vi "HFRR ADV v04.vi"() -> ()   [LabVIEW 2025] (continued)
                n419 = Array To Spreadsheet String(delimiter (Tab)=";", array=w743, 3:"" ("format string")) -> (spreadsheet string=w745:string)
                "String 9" <- w745
                n420 = Concatenate Strings("FF ( V ); DP( mincron ) " ("character string"), "\r") -> (w758:string)
                n421 = local read "file count"() -> (w741:i32)
                n422 = local read "FILE 2"() -> (w746:string)
                n423 = local write "save dpt"(FALSE ("Hold 3")) -> ()
                n424 = Number To Decimal String(number=w741) -> (decimal integer string=w747:string)  [unwired: 1 in]
                n425 = Concatenate Strings(w746, w747) -> (w739:string)
                n426 = Concatenate Strings("C:\\LAB-IQ-NXT\\data" ("Substring"), w739) -> (w754:string)
                n427 = Concatenate Strings(w754, ".dpf" ("Substring")) -> (w752:string)
                n428 = Add(x=1, y=w741) -> (x+y=w742:i32)
                n429 = local write "file count"(w742) -> ()
                n430 = String To Path(string=w752) -> (path=w750:path)
                n431 = call <vilib>:"Write Characters To File.vi"("append to file? (new file:F)"=FALSE, "character string"=w758, "file path (dialog if empty)"=w750) -> ("new file path (Not A Path if cancelled)"=w755:path)  [unwired: 2 in]
                n432 = call <vilib>:"Write Characters To File.vi"("append to file? (new file:F)"=TRUE, "character string"=w745, "file path (dialog if empty)"=w755) -> ()  [unwired: 2 in, 1 out]
              }
            }
          }
          frame #5 {
            n433 = case shown="True" "Hold 4" {
              frame False {
              }
              frame True {
                n434 = File Dialog(6:"*.dpf" ("pattern"), 11:path "C:/LAB-IQ-NXT" ("start path")) -> (0:w765:errorcluster, 3:w780:path)  [unwired: 5 in, 2 out]
                n435 = Unbundle(w765) -> ()  [unwired: 3 out]
                n436 = call <vilib>:"Read Characters From File.vi"("file path (dialog if empty)"=w780) -> ("character string"=w770:string)  [unwired: 5 in, 3 out]
                n437 = Spreadsheet String To Array(delimiter (Tab)=";", format string="%S", spreadsheet string=w770, array type (2D Dbl)=string[][] []) -> (array=w774:string[][])
                n438 = for {
                  tunnel: w774 -> [w784] mode=indexing
                  tunnel: [w783] -> w775 mode=indexing
                  n439 = for {
                    tunnel: w784 -> [w786] mode=indexing
                    tunnel: [w785] -> w783 mode=indexing
                    n440 = call <vilib>:"Trim Whitespace.vi"("string"=w786) -> ("trimmed string"=w785:string)  [unwired: 1 in]
                  }
                }
                n441 = Fract/Exp String To Number(string=w775) -> (number=w777:dbl[][])  [unwired: 3 in, 1 out]
                n442 = Array Subset(array=w777, index (row)=1 ("index (col)")) -> (w779:dbl[][])  [unwired: 3 in]
                n443 = Index Array(array=w779, index (col) #1=0 ("disabled index (col)"), index (col) #2=1 ("disabled index (col)")) -> (element #1=w768:dbl[], element #2=w767:dbl[])  [unwired: 2 in]
                n444 = Build Array(w768, w767) -> (→"Waveform Graph":dbl[][])
              }
            }
          }
        }
      }
      frame Error {
        w802 = u16 0 items=["None", "XON/XOFF", "RTS/CTS", "XON/XOFF & RTS/CTS", "DTR/DSR", "XON/XOFF & DTR/DSR"] ("flow control (0:none)  2")
        w800 = u16 10 items=["1.0"=10, "1.5"=15, "2.0"=20] ("stop bits 2")
        w798 = u16 0 items=["None", "Odd", "Even", "Mark", "Space"] ("parity 2")
        w799 = u32 10000  # timeout (10sec)
        n445 = VISA Close(VISA resource name=w794, error in (no error)=w791) -> (error out=w795:errorcluster)
        n446 = local read "Com Port 1"() -> (w787:refnum<visa-resource-name>)
        n447 = call <vilib>:"Clear Errors.vi"("error in (no error)"=w795) -> ("error out"=w792:errorcluster)  [unwired: 5 in, 1 out]
        n448 = local write "Sps 3"(0.0 ("Sps 4")) -> ()
        n449 = call-poly "VISA Configure Serial Port"("VISA resource name"=w787, "timeout (10sec)"=w799, "baud rate (9600)"=u32 250000 ("baud rate  2"), "data bits (8)"=u16 8 ("data bits  2"), "parity (0:none)"=w798, "error in (no error)"=w792, "stop bits (10: 1 bit)"=w800, "flow control (0:none)"=w802) -> ("VISA resource name out"=w803:refnum<visa-resource-name>, "error out"=w804:errorcluster)  [unwired: 6 in]
        n450 = flat-sequence {
          tunnel: w803 -> [w806]
          tunnel: w804 -> [w805]
          tunnel: [w806] -> w796
          tunnel: [w805] -> w788
          frame #0 {
            n451 = Wait (ms)(milliseconds to wait=u32 50) -> ()  [unwired: 1 out]
          }
        }
        "Residual Uno" <- ""
        "Port 1 Error" <- w788
      }
    }
    n452 = local read "Port 1a"() -> (w449:bool)
    n453 = local read "Port 3"() -> (w450:bool)
    n454 = Or(x=w450, y=w449) -> (x .or. y?=w452:bool)
    n455 = case shown="False" w452 {
      frame False {
        w463 = FALSE ("Visible")
        n456 = property on="Port 1a" class="Bool (strict)"("Visible"=w463) -> ()  [unwired: 2 in, 2 out]
        n457 = property on="Port 3" class="Bool (strict)"("Visible"=w463) -> ()  [unwired: 2 in, 2 out]
      }
      frame True {
        w464 = TRUE ("Visible")
        n458 = property on="Port 1a" class="Bool (strict)"("Visible"=w464) -> ()  [unwired: 2 in, 2 out]
        n459 = property on="Port 3" class="Bool (strict)"("Visible"=w464) -> ()  [unwired: 2 in, 2 out]
      }
    }
    n460 = local read "EXIT"() -> (w454:bool)
    "Error Uno" <- w448
  }
  n461 = while {
    tunnel: w43 -> [_]
    tunnel: [w829] -> _
    tunnel: w15 -> [_]
    tunnel: ["EXIT"] -> w40
    i -> [w829]
    stop <- "EXIT" stop-if-true
    # "C:\\LAB-IQ-NXT\\Scar View.exe"
    n462 = local read "RUN"() -> (w827:bool)
    n463 = local read "EDIT 2"() -> (w814:bool)
    n464 = case shown="False" w827 {
      frame False {
        n465 = local read "stopT"() -> (w1697:bool)
        n466 = case shown="True" w1697 {
          frame False {
          }
          frame True {
            w1698 = FALSE
            n467 = local write "st enable"(w1698) -> ()
            n468 = local write "stopT"(w1698) -> ()
          }
        }
      }
      frame True {
        "stopT" <- TRUE
      }
    }
    n469 = case shown="True" w814 {
      frame False {
        n470 = local write "Password 2"("" ("Password")) -> ()
        n471 = property on="Password 2" class="Str"("Visible"=FALSE) -> ()  [unwired: 2 in, 2 out]
      }
      frame True {
        n472 = property on="Password 2" class="Str"("Visible"=TRUE) -> ()  [unwired: 2 in, 2 out]
        n473 = Equal?(x="Password 2", y="HFRR1234") -> (x = y?=w842:bool)
        n474 = case shown="True" w842 {
          tunnel: "Password 2" -> [w845 _]
          frame False {
            n475 = String Length(string=w845) -> (length=w846:i32)
            n476 = Greater Than 0?(x=w846) -> (x > 0?=w844:bool)
            n477 = case shown="False" w844 {
              frame False {
                n478 = property on="Password 2" class="Str"("Caption.Text"="Password (Advance Setting)") -> ()  [unwired: 2 in, 2 out]
              }
              frame True {
                n479 = property on="Password 2" class="Str"("Caption.Text"="Incorrect Password!") -> ()  [unwired: 2 in, 2 out]
              }
            }
          }
          frame True {
            n480 = local write "Password 2"("" ("Password")) -> ()
            n481 = local write "Main Tab"(T2."Advance" ("Main Tab")) -> ()
            n482 = local write "EDIT 2"(FALSE ("EDIT 2")) -> ()
          }
        }
      }
    }
    n483 = Wait (ms)(milliseconds to wait=u32 50) -> ()  [unwired: 1 out]
    n484 = case shown="True" "EDIT 3" {
      frame False {
      }
      frame True {
        n485 = local write "EDIT 3"(FALSE ("EDIT 3")) -> ()
        n486 = local write "Main Tab"(T2."About" ("Main Tab")) -> ()
      }
    }
    n487 = local read "Re-Initialise"() -> (w812:bool)
    n488 = case shown="True" w812 {
      frame False {
      }
      frame True {
        n489 = local write "Re-Initialise"(FALSE ("Re-Initialise")) -> ()
      }
    }
    n490 = case shown="\"CEC F-096-A-06\"" "TEST STANDARD" {
      tunnel: [2.0 ("Set Temp") 0.0 ("Set Temp") 2.0 ("Set Temp") 0.0 ("Set Temp")] -> w815
      frame "ASTM D6079", Default {
        # "astm hide"
        n491 = local write "Set Hz"(50.0 ("Hz")) -> ()
        n492 = local write "Set Strk"(1.0 ("Set Strk")) -> ()
        n493 = local write "Set Rh"(53.0 ("Set Rh")) -> ()
        n494 = local write "Set Temp"(60.0 ("Set Temp")) -> ()
        n495 = local write "test time"(75.0 ("test time")) -> ()
        n496 = local write "NORMAL LOAD"(2.0 ("NORMAL LOAD")) -> ()
        "Test Standard" <- "ASTM D6079" ("Test Standard 2")
      }
      frame "ISO 12156" {
        n497 = local write "Set Hz"(50.0 ("Hz")) -> ()
        n498 = local write "Set Rh"(53.0 ("Set Rh")) -> ()
        n499 = local write "Set Strk"(1.0 ("Set Strk")) -> ()
        n500 = local write "test time"(75.0 ("test time")) -> ()
        n501 = local write "Set Temp"(60.0 ("Set Temp")) -> ()
        n502 = local write "NORMAL LOAD"(2.0 ("NORMAL LOAD")) -> ()
      }
      frame "CEC F-096-A-06" {
        n503 = local write "Set Strk"(1.0 ("Set Strk")) -> ()
        n504 = local write "Set Hz"(50.0 ("Hz")) -> ()
        n505 = local write "Set Rh"(53.0 ("Set Rh")) -> ()
        n506 = local write "Set Temp"(60.0 ("Set Temp")) -> ()
        n507 = local write "test time"(75.0 ("test time")) -> ()
        n508 = local write "NORMAL LOAD"(2.0 ("NORMAL LOAD")) -> ()
      }
      frame "Custom" {
      }
    }
    n509 = local read "OPEN 6"() -> (w811:bool)
    n510 = local read "service 3"() -> (w809:bool)
    n511 = Or(x=w811, y=w809) -> (x .or. y?=w810:bool)
    n512 = local read "RUN"() -> (w824:bool)
    n513 = case shown="True" w810 {
      selector: w810 -> [_ w834]
      frame False {
      }
      frame True {
        n514 = Not(x=w834) -> (.not. x?=w830:bool)
        n515 = local write "service 3"(w830) -> ()
        n516 = local write "OPEN 6"(w830) -> ()
        n517 = call <vilib>:"System Exec.vi"("wait until completion? (T)"=TRUE, "command line"="C:\\LAB-IQ-NXT\\Scar View.exe") -> ("error out"=→"error out 5":errorcluster)  [unwired: 6 in, 3 out]
      }
    }
    n518 = case shown="True" w824 {
      frame False {
      }
      frame True {
        n519 = local read "Main Tab"() -> (w1695:T2)
        n520 = case shown="\"Compare Files\"" w1695 {
          frame "Acquire", Default {
          }
          frame "Compare Files" {
            n521 = local write "Main Tab"(T2."Acquire" ("Main Tab")) -> ()
          }
          frame "About" {
          }
        }
      }
    }
    n522 = local read "Main Tab"() -> (w808:T2)
    n523 = case shown="\"Compare Files\"" w808 {
      tunnel: [T15."Acquire" ("Main Tab") T16."   COMPARE   FILES " ("Tab Control") T17."PRINT REPORT" ("Tab Control")] -> w822
      frame "Acquire", Default {
      }
      frame "Compare Files" {
      }
      frame "About" {
      }
    }
    n524 = property on="SetTemp" class="DigNum (strict)"("Disabled"=w815) -> ()  [unwired: 2 in, 2 out]
    n525 = case shown="2" w822 {
      frame 0, Default {
        w1836 = 0.2 ("y")
        w1841 = 1.0 ("y")
        w1842 = 0.8 ("y")
        # "Elapsed time\ncof\nstroke\nAir temp\nTemp\nHumidity"
        n526 = case shown="True" "Save & Continue" {
          frame False {
          }
          frame True {
            "acq 2" <- TRUE ("acq 2")
          }
        }
        n527 = disable-structure shown="Disabled" {
          frame Disabled {
            n528 = case shown="False" {
              selector: _ -> [_ _]
              frame False {
              }
              frame True {
                n529 = local read "zflag 2"() -> (w1874:dbl)
                n530 = local read "yflag"() -> (w1876:dbl)
                n531 = Equal?(x=w1874, y=3.0 ("tflag")) -> (x = y?=w1877:bool)
                n532 = Equal?(x=w1876, y=2.0 ("tflag")) -> (x = y?=w1878:bool)
                n533 = And(x=w1878, y=w1877) -> (x .and. y?=w1872:bool)
                n534 = case shown="True" w1872 {
                  frame False {
                  }
                  frame True {
                    w1903 = 0.0 ("zflag")
                    n535 = local read "SEN.RUN HRS"() -> (w1889:dbl)
                    n536 = local read "SENSOR TIME"() -> (w1887:dbl)
                    n537 = local read "Total No. of Tests"() -> (w1890:dbl)
                    n538 = Delete(path (use dialog)=path "C:/LAB-IQ-NXT/WO 2449 TRH.sig" ("file path (dialog if empty)")) -> (deleted path=w1897:path)  [unwired: 4 in, 2 out]
                    n539 = Add(x=w1887, y=w1889) -> (x+y=w1888:dbl)
                    "SEN.RUN HRS" <- w1888
                    n540 = Number To Decimal String(number=w1888) -> (decimal integer string=w1894:string)  [unwired: 1 in]
                    n541 = call <vilib>:"compatOverwrite.vi"("overwrite (F)"=TRUE) -> ("overwrite?"=w1883:T20)
                    n542 = Delete(path (use dialog)=path "C:/LAB-IQ-NXT/WO 2449 TT.sig" ("file path (dialog if empty)")) -> (deleted path=w1902:path)  [unwired: 4 in, 2 out]
                    n543 = Open/Create/Replace File(file path (use dialog)=w1897, operation (0:open)=w1883) -> (refnum out=w1884:refnum<file>, error out=w1885:errorcluster)  [unwired: 4 in, 1 out]
                    n544 = Number To Decimal String(number=w1890) -> (decimal integer string=w1898:string)  [unwired: 1 in]
                    n545 = Deny Access(4:w1885, 6:T18."deny none" ("deny mode (2)"), 7:w1884) -> (3:w1893:refnum<file>)  [unwired: 1 out]
                    n546 = call <vilib>:"compatOverwrite.vi"("overwrite (F)"=TRUE) -> ("overwrite?"=w1879:T20)
                    n547 = Write to Binary File(file (use dialog)=w1893, data=w1894, 5:FALSE ("prepend array or string size? (T)")) -> ()  [unwired: 3 in, 3 out]
                    n548 = Open/Create/Replace File(file path (use dialog)=w1902, operation (0:open)=w1879) -> (refnum out=w1880:refnum<file>, error out=w1881:errorcluster)  [unwired: 4 in, 1 out]
                    n549 = Deny Access(4:w1881, 6:T18."deny none" ("deny mode (2)"), 7:w1880) -> (3:w1901:refnum<file>)  [unwired: 1 out]
                    n550 = local write "zflag"(w1903) -> ()
                    n551 = local write "zflag 2"(w1903) -> ()
                    n552 = Write to Binary File(file (use dialog)=w1901, data=w1898, 5:FALSE ("prepend array or string size? (T)")) -> ()  [unwired: 3 in, 3 out]
                  }
                }
              }
            }
          }
          frame Enabled {
          }
        }
        n553 = case shown="True" "Save & Continue" {
          frame False {
          }
          frame True {
            n554 = while {
              tunnel: "0123456789abcdefghijklmnopqrstuvwxyzABCDEFGHIJKLMNOPQRSTUVWXYZ" ("string 2") -> [w1963]
              shift-right: [w1961] -> w1956
              shift-left: "" -> [w1960]
              i -> [w1970]
              stop <- w1969 stop-if-true
              n555 = Random Number (0-1)() -> (number: 0 to 1=w1964:dbl)
              n556 = Multiply(x=w1964, y=62.0) -> (x*y=w1966:dbl)
              n557 = Decrement(x="Length") -> (x-1=w1959:i16)
              n558 = To Word Integer(number=w1966) -> (16bit integer=w1967:i16)
              n559 = String Subset(string=w1963, offset (0)=w1967, length (rest)=1 ("length (rest)")) -> (substring=w1962:string)
              n560 = Greater Or Equal?(x=w1970, y=w1959) -> (x >= y?=w1969:bool)
              n561 = Concatenate Strings(w1962, w1960) -> (w1961:string)
            }
            n562 = local write "UUID"(w1956) -> ()
          }
        }
        n563 = case shown="True" "Save & Continue" {
          frame False {
          }
          frame True {
            n564 = local read "Operator ID"() -> (w2248:string)
            n565 = local read "FILE"() -> (w2255:string)
            n566 = String Length(string=w2248) -> (length=w2249:i32)
            n567 = String Length(string=w2255) -> (length=w2253:i32)
            n568 = Greater?(x=w2249, y=0) -> (0:w2247:bool)
            n569 = Greater?(x=w2253, y=0) -> (0:w2252:bool)
            n570 = And(x=w2252, y=w2247) -> (x .and. y?=w2251:bool)
            n571 = case shown="True" w2251 {
              frame False {
                n572 = stacked-sequence {
                  frame #0 {
                    n573 = One Button Dialog(message="Please Enter a File Name and Operator ID to save data !", button name ("OK")="Ok") -> ()  [unwired: 1 out]
                  }
                  frame #1 {
                    n574 = local write "Save & Continue"(FALSE ("OK Button")) -> ()
                  }
                }
                n575 = local write "Save & Continue"(FALSE ("OK Button")) -> ()
              }
              frame True {
                n576 = stacked-sequence {
                  frame #0 {
                    (unwired) ")!" ("string")
                    (unwired) ")" ("string")
                    w2260 = dbl[] [] ("History Data")
                    w2264 = "\r"
                    # "C:\\WinDucom\\Data\\"
                    # "C:\\LAB-IQ-NXT\\data"
                    n577 = local read "Batch Ref Num :"() -> (w2262:string)
                    n578 = local read "NORMAL LOAD"() -> (w2281:dbl)
                    n579 = local read "Fuel Discription :"() -> (w2275:string)
                    n580 = Multiply(x=w2281, y=1.0) -> (x*y=w2280:dbl)
                    n581 = Number To Fractional String(number=w2280, width (-)=i16 5, precision (6)=i16 2) -> (F-format string=w2289:string)  [unwired: 1 in]
                    n582 = Concatenate Strings(w2275) -> (w2276:string)
                    n583 = local read "Remarks :"() -> (w2274:string)
                    n584 = property on="Electrical Contact Resistance ( % )" class="WFChart (strict)"("History Data"=w2260) -> ()  [unwired: 2 in, 2 out]
                    n585 = Get Date/Time String(date format (0)=enum16{"short", "long", "abbreviated"}."short") -> (date string=w2300:string, time string=w2297:string)  [unwired: 2 in]
                    n586 = property on="Coefficient of Friction" class="WFChart (strict)"("History Data"=w2260) -> ()  [unwired: 2 in, 2 out]
                    n587 = property on="Frictional Force ( N )" class="WFChart (strict)"("History Data"=w2260) -> ()  [unwired: 2 in, 2 out]
                    n588 = Concatenate Strings(w2262) -> (w2261:string)
                    n589 = Concatenate Strings(w2274, "," ("string")) -> (w2273:string)
                    n590 = Concatenate Strings("Load :- " ("Substring"), w2289, " N ," ("Substring")) -> (w2288:string)
                    n591 = local read "String 41"() -> (w2266:string)
                    n592 = local read "FILE"() -> (w2308:string)
                    n593 = Concatenate Strings("(" ("Substring"), w2300, ")" ("Substring"), w2297) -> (w2268:string)
                    "concatenated string" <- w2268
                    n594 = Concatenate Strings("C:\\LAB-IQ-NXT\\data\\" ("string"), w2308) -> (w2307:string)
                    n595 = Concatenate Strings("tested by") -> (w2270:string)
                    n596 = Concatenate Strings(w2307, ".duf" ("Substring")) -> (w2304:string)
                    n597 = Concatenate Strings(w2307, ".dgf" ("Substring")) -> (w2303:string)
                    n598 = String To Path(string=w2303) -> (path=w2301:path)
                    n599 = String To Path(string=w2304) -> (path=w2278:path)
                    n600 = Concatenate Strings(w2266, w2264, "Fuel Discription :-" ("Substring"), w2276, w2264, w2288, w2264, "Batch Ref Num :-" ("Substring"), w2261, w2264, " Remarks :- " ("Substring"), w2273, w2264, " Date :- " ("Substring"), w2268, w2264, "Tested By :-" ("Substring"), w2270) -> (w2282:string)
                    "REMARKS" <- w2282
                    n601 = local write "clk"(0.0 ("clk")) -> ()
                    n602 = local write "speedop"(0.0 ("PIDclk 2")) -> ()
                    n603 = Concatenate Strings("  TIME;      COF;       STROKE;     AIR TEMP;  TEMP;  HUMIDITY;  ECR; PID-OUT; FREQUENCY" ("Substring"), "\r") -> (w2284:string)
                    n604 = call <vilib>:"Write Characters To File.vi"("append to file? (new file:F)"=FALSE, "character string"=w2284, "file path (dialog if empty)"=w2301) -> ()  [unwired: 2 in, 1 out]
                    n605 = call <vilib>:"Write Characters To File.vi"("append to file? (new file:F)"=FALSE, "character string"=w2282, "file path (dialog if empty)"=w2278) -> ()  [unwired: 2 in, 1 out]
                  }
                  frame #1 {
                    n606 = local write "autostrtflg"(TRUE ("autostrtflg")) -> ()
                    n607 = local write "Main Tab"(T2."Acquire" ("Main Tab")) -> ()
                    n608 = local write "Save & Continue"(FALSE ("OK")) -> ()
                    n609 = local write "STOP 3"(FALSE ("STOP")) -> ()
                    n610 = One Button Dialog(message="Please ensure sample is mounted properly and machine is ready in all aspects for testing !", button name ("OK")="Ok") -> ()  [unwired: 1 out]
                    n611 = property on="Save & Continue" class="Bool (strict)"("Visible"=FALSE ("OK")) -> ()  [unwired: 2 in, 2 out]
                    n612 = property on="STOP 3" class="Bool (strict)"("Visible"=TRUE) -> ()  [unwired: 2 in, 2 out]
                    n613 = Get Date/Time In Seconds() -> (seconds since 1Jan1904=w2314:timestamp)
                    n614 = local write "Cycles elapsed"(0 ("Cycles elapsed")) -> ()
                    n615 = To Double Precision Float(number=w2314) -> (double precision float=w2313:dbl)
                    n616 = local write "cyclecount"(0 ("cyclecount")) -> ()
                    n617 = local write "acq timer"(w2313) -> ()
                    n618 = local write "Save"(FALSE ("Save")) -> ()
                  }
                }
              }
            }
          }
        }
        n619 = case shown="True" "STOP 3" {
          frame False {
          }
          frame True {
            w2240 = "" ("Sample ID :")
            (unwired) FALSE ("Visible")
            n620 = local write "Save & Continue"(FALSE ("OK Button")) -> ()
            n621 = local write "STOP 3"(FALSE ("STOP")) -> ()
            n622 = local write "clk"(0.0 ("clk")) -> ()
            n623 = local write "RUN"(FALSE ("OK Button 2")) -> ()
            n624 = property on="Save & Continue" class="Bool (strict)"("Visible"=TRUE) -> ()  [unwired: 2 in, 2 out]
            n625 = property on="STOP 3" class="Bool (strict)"("Visible"=FALSE) -> ()  [unwired: 2 in, 2 out]
            n626 = property on="STOP 2" class="Bool (strict)"("Disabled"=u8 0) -> ()  [unwired: 2 in, 2 out]
            n627 = local write "Fuel Discription :"(w2240) -> ()
            n628 = local write "Remarks :"(w2240) -> ()
            n629 = local write "tested by"(w2240) -> ()
            n630 = local write "FILE"(w2240) -> ()
            n631 = local write "Batch Ref Num :"(w2240) -> ()
          }
        }
        n632 = local read "AIR TEMP"() -> (w1810:dbl)
        n633 = local read "run replace"() -> (w1848:bool)
        n634 = Greater Or Equal?(x=w1810, y=15.0) -> (x >= y?=w1811:bool)
        "powstat" <- w1811
        n635 = local read "acq 2"() -> (w1847:bool)
        n636 = And(x=w1847, y=w1848) -> (x .and. y?=w1846:bool)
        n637 = local read "run replace"() -> (w1849:bool)
        n638 = case shown="True" w1846 {
          frame False {
            n639 = local write "tfalg"(0.0 ("tfalg")) -> ()
          }
          frame True {
            n640 = local read "tfalg"() -> (w1947:dbl)
            n641 = Equal?(x=w1947, y=0.0) -> (x = y?=w1948:bool)
            n642 = case shown="True" w1948 {
              frame False {
              }
              frame True {
                n643 = local read "Total No. of Tests"() -> (w1951:dbl)
                n644 = Increment(x=w1951) -> (x+1=w1950:dbl)
                n645 = local write "Total No. of Tests"(w1950) -> ()
                n646 = local write "tfalg"(1.0 ("tfalg")) -> ()
                n647 = local write "acq 2"(FALSE ("acq 2")) -> ()
                n648 = Wait (ms)(milliseconds to wait=u32 200) -> ()  [unwired: 1 out]
              }
            }
          }
        }
        n649 = case shown="False" w1849 {
          frame False {
            n650 = local read "zflag"() -> (→"zflag 2":dbl)
            n651 = local write "FLAG 4"(0.0 ("FLAG")) -> ()
            n652 = local write "yflag"(2.0 ("tflag")) -> ()
          }
          frame True {
            n653 = local write "zflag"(3.0 ("zflag")) -> ()
            n654 = local write "yflag"(1.0 ("tflag")) -> ()
          }
        }
        n655 = property on="STOP 3" class="Bool (strict)"() -> ("Visible"=w1851:bool)  [unwired: 2 in, 2 out]
        n656 = case shown="True" w1851 {
          tunnel: [FALSE ("Visible") TRUE ("Visible")] -> w1861
          frame False {
          }
          frame True {
          }
        }
        n657 = property on="RUN" class="Bool (strict)"("Visible"=w1861) -> ()  [unwired: 2 in, 2 out]
        n658 = property on="Save & Continue" class="Bool (strict)"() -> ("Visible"=w1864:bool)  [unwired: 2 in, 2 out]
        n659 = local read "RUN"() -> (w1845:bool)
        n660 = case shown="True" w1845 {
          frame False {
            n661 = local read "Rt 3"() -> (w1929:bool)
            n662 = case shown="True" w1929 {
              frame False {
              }
              frame True {
                n663 = local write "Json End Flg"(TRUE ("Upld AR 2")) -> ()
                n664 = local write "Rt 3"(FALSE ("Rt 3")) -> ()
              }
            }
            "Rt" <- TRUE ("Rt")
            "Rt 2" <- FALSE ("Rt")
          }
          frame True {
            n665 = local read "Rt"() -> (w1936:bool)
            n666 = case shown="True" w1936 {
              frame False {
              }
              frame True {
                w1937 = TRUE ("Upld AR 2")
                n667 = local write "Rt"(FALSE ("Rt")) -> ()
                n668 = local write "Upld AR"(w1937) -> ()
                n669 = local write "Json St Flg"(w1937) -> ()
              }
            }
            n670 = local write "Rt 2"(TRUE ("Rt 2")) -> ()
            "Rt 3" <- TRUE ("Rt 3")
          }
        }
        n671 = Not(x=w1864) -> (.not. x?=w1863:bool)
        n672 = case shown="True" w1845 {
          frame False {
            n673 = local write "run replace"(FALSE ("run replace")) -> ()
          }
          frame True {
            "run replace" <- TRUE ("run replace")
          }
        }
        n674 = And(x=w1863, y=w1851) -> (x .and. y?=w1860:bool)
        "Test Status 2" <- w1860
        n675 = case shown="True" w1860 {
          tunnel: w1811 -> [_ w2002]
          frame False {
            w2000 = 0.0 ("output")
            n676 = local write "Frequency ( Hz )"(w2000) -> ()
            n677 = local write "PID-out"(w2000) -> ()
            n678 = local write "Heater Button"(FALSE ("Heater Button")) -> ()
          }
          frame True {
            n679 = case shown="False" w2002 {
              frame False {
                n680 = stacked-sequence {
                  frame #0 {
                    n681 = local write "RUN"(FALSE ("OK Button 2")) -> ()
                  }
                  frame #1 {
                    n682 = property on="RUN" class="Bool (strict)"("Visible"=FALSE) -> ()  [unwired: 2 in, 2 out]
                  }
                }
              }
              frame True {
              }
            }
            n683 = stacked-sequence {
              frame #0 {
                n684 = Not(x="Engage") -> (.not. x?=w2010:bool)
                n685 = case shown="True" "RUN" {
                  tunnel: [w2028 w2036] -> w2006
                  frame False {
                    w2028 = 0.0
                    n686 = local write "Reinit PID"(TRUE) -> ()
                    n687 = property on="Stroke 2" class="DigNum (strict)"("Visible"=FALSE) -> ()  [unwired: 2 in, 2 out]
                    n688 = property on="Stroke" class="DigNum (strict)"("Visible"=TRUE) -> ()  [unwired: 2 in, 2 out]
                    n689 = local write "String 14"("Test will autostart once parameters reach the set value." ("String 14")) -> ()
                    n690 = local write "Old Pid Val"(w2028) -> ()
                  }
                  frame True {
                    n691 = local read "PID Ref"() -> (w2047:bool)
                    n692 = property on="STOP 2" class="Bool (strict)"("Disabled"=u8 2) -> ()  [unwired: 2 in, 2 out]
                    n693 = case shown="True" w2047 {
                      tunnel: [w2048 w2064] -> w2046
                      frame False {
                        n694 = local read "Old Pid Val"() -> (w2048:dbl)
                      }
                      frame True {
                        n695 = local read "Set Hz"() -> (w2057:dbl)
                        n696 = Add(x=w2057, y=-10.0 ("Offset")) -> (x+y=w2075:dbl)
                        n697 = local read "Frequency"() -> (w2068:dbl)
                        n698 = Add(x=w2057, y=-10.0) -> (x+y=w2067:dbl)
                        n699 = Add(x=w2057, y=10.0) -> (x+y=w2066:dbl)
                        n700 = Multiply(x=w2075, y=0.1 ("Gain")) -> (x*y=w2054:dbl)
                        n701 = Add(x=w2054, y=1.5) -> (x+y=w2052:dbl)
                        n702 = local read "SPEED OUT:"() -> (w2076:dbl)
                        n703 = In Range and Coerce(upper limit=w2066, x=w2068, lower limit=w2067) -> (coerced(x)=w2056:dbl)  [unwired: 1 out]
                        n704 = Multiply(x=w2052, y=w2076) -> (x*y=w2051:dbl)
                        n705 = Multiply(x=w2051, y=0.8) -> (x*y=w2050:dbl)
                        n706 = local read "Elapsed time"() -> (w2061:dbl)
                        n707 = Or(x="Reinit PID", y="Reinit PID") -> (x .or. y?=w2065:bool)
                        n708 = call-poly <vilib>:"PID.vi"("reinitialize? (F)"=w2065, "output range"=cluster{"output high":dbl, "output low":dbl} {"output high"=1.0, "output low"=-1.0}, "PID gains"=T10 {"proportional gain (Kc)"=0.0005, "integral time (Ti, min)"=0.001, "derivative time (Td, min)"=0.0} ("Motor PID"), "process variable"=w2056, "setpoint"=w2057) -> ("output"=w2055:dbl)  [unwired: 5 in, 1 out]
                        n709 = Greater?(x=w2061, y=0.05) -> (0:w2060:bool)
                        n710 = case shown="True" w2060 {
                          tunnel: w2055 -> [_ w2078]
                          tunnel: [0.0 ("output") w2078] -> w2058
                          frame False {
                          }
                          frame True {
                            n711 = local write "Reinit PID"(FALSE ("Reinit PID")) -> ()
                          }
                        }
                        n712 = Add(x=w2050, y=w2058) -> (x+y=w2063:dbl)
                        n713 = flat-sequence {
                          tunnel: [w2081] -> w2064
                          tunnel: w2063 -> [w2081]
                          frame #0 {
                            n714 = local write "PID Ref"(FALSE ("PID Ref")) -> ()
                          }
                        }
                      }
                    }
                    "Old Pid Val" <- w2046
                    n715 = local read "Set Hz"() -> (w2043:dbl)
                    n716 = local read "Freq"() -> (w2035:dbl)
                    n717 = call <vilib>:"Uniform White Noise Waveform.vi"() -> ("signal out"=w2042:waveform(dbl))  [unwired: 10 in, 1 out]
                    n718 = property on="RUN" class="Bool (strict)"("Visible"=TRUE) -> ()  [unwired: 2 in, 2 out]
                    n719 = Add(x=w2043, y=w2042) -> (x+y=w2041:waveform(dbl))
                    n720 = property on="Stroke 2" class="DigNum (strict)"("Visible"=TRUE) -> ()  [unwired: 2 in, 2 out]
                    n721 = property on="Stroke" class="DigNum (strict)"("Visible"=FALSE) -> ()  [unwired: 2 in, 2 out]
                    n722 = Multiply(x=w2041, y=ext 0.1) -> (x*y=w2037:waveform(ext))
                    n723 = Multiply(x=w2035, y=0.9) -> (x*y=w2038:dbl)
                    n724 = local write "String 14"(" Running....." ("String 14")) -> ()
                    n725 = Add(x=w2037, y=w2038) -> (x+y=w2036:waveform(ext))
                  }
                }
                n726 = call "Elapsed Time"("Time Target (s)"="Countdown", "Reset"=w2010) -> ("Elapsed Time (s)"=w2015:dbl, "Time has Elapsed"=w2013:bool)  [unwired: 10 in, 6 out]
                "Countdown 2" <- w2015
                n727 = Subtract(x=w2015, y=2.0) -> (x-y=w2018:dbl)
                n728 = Less?(x=w2018, y="Countdown") -> (x < y?=w2016:bool)
                n729 = And(x=w2016, y=w2013) -> (x .and. y?=w2012:bool)
                n730 = case shown="True" w2012 {
                  frame False {
                  }
                  frame True {
                    (unwired) dbl[] [] ("History Data")
                    n731 = local read "Humidity ( %RH )"() -> (→"Rh Before":dbl)
                    n732 = local write "RUN"(TRUE ("RUN")) -> ()
                    n733 = local write "Engage"(FALSE ("Engage")) -> ()
                  }
                }
                n734 = local read "clk"() -> (w2023:dbl)
                n735 = local read "Save"() -> (w2019:bool)
                n736 = Equal?(x=w2023, y=0.0) -> (x = y?=w2020:bool)
                n737 = And(x=w2020, y=w2019) -> (x .and. y?=w2021:bool)
                n738 = case shown="True" w2021 {
                  frame False {
                  }
                  frame True {
                    n739 = Get Date/Time In Seconds() -> (seconds since 1Jan1904=w2084:timestamp)
                    n740 = To Double Precision Float(number=w2084) -> (double precision float=w2082:dbl)
                    n741 = local write "act save time"(w2082) -> ()
                    n742 = local write "acq timer"(w2082) -> ()
                    n743 = local write "clk"(10.0 ("clk")) -> ()
                  }
                }
                n744 = local read "Test \nStatus"() -> (w2008:bool)
                n745 = Select(t=w2006, s=w2008, f=0.0) -> (s? t:f=w2007:dbl)
                n746 = local write "Frequency ( Hz )"(w2007) -> ()
                n747 = local write "Freq"(w2007) -> ()
              }
              frame #1 {
                w2107 = 1000000.0 ("x")
                # "Elapsed time\ncof\nstroke\nAir temp\nTemp\nHumidity"
                # "acq timer\n\nact save time"
                # "convert to microseconds"
                n748 = local read "COUNT"() -> (w2090:i32)
                n749 = Greater Or Equal?(x=w2090, y=250) -> (x >= y?=w2089:bool)
                n750 = case shown="True" w2089 {
                  frame False {
                    n751 = local read "COUNT"() -> (w2111:i32)
                    n752 = Increment(x=w2111) -> (x+1=w2112:i32)
                    n753 = local write "COUNT"(w2112) -> ()
                  }
                  frame True {
                    n754 = local write "COUNT"(0 ("COUNT")) -> ()
                  }
                }
                n755 = local read "Samplingtime 2"() -> (w2088:dbl)
                n756 = local read "act save time"() -> (w2105:dbl)
                n757 = Get Date/Time In Seconds() -> (seconds since 1Jan1904=w2110:timestamp)
                n758 = To Double Precision Float(number=w2110) -> (double precision float=w2099:dbl)
                n759 = local read "acq timer"() -> (w2109:dbl)
                n760 = Add(x=w2105, y=w2088) -> (x+y=w2104:dbl)
                n761 = Greater Or Equal?(x=w2099, y=w2104) -> (x >= y?=w2087:bool)
                n762 = Subtract(x=w2099, y=w2109) -> (x-y=w2101:dbl)
                n763 = local read "Rate"() -> (w2103:dbl)
                n764 = Divide(x=w2107, y=w2103) -> (x/y=w2108:dbl)
                n765 = Divide(x=w2108, y=w2107) -> (x/y=w2106:dbl)
                n766 = local read "Save"() -> (w2102:bool)
                n767 = And(x=w2087, y=w2102) -> (x .and. y?=w2100:bool)
                n768 = case shown="True" w2100 {
                  tunnel: w2099 -> [_ w2185]
                  tunnel: [FALSE ("Boolean 2") TRUE ("Boolean 2")] -> _
                  frame False {
                  }
                  frame True {
                    w2154 = ";" ("Substring")
                    # "Pid out/\nFreq response value"
                    n769 = local write "act save time"(w2185) -> ()
                    n770 = local read "Set Strk"() -> (w2153:dbl)
                    n771 = local read "Stroke"() -> (w2144:dbl)
                    n772 = local read "FF 2"() -> (w2139:dbl)
                    "Frictional Force ( N )" <- w2139
                    "Frictional Force ( N )" <- w2139
                    n773 = Subtract(x=w2144, y=w2153) -> (x-y=w2150:dbl)
                    n774 = local read "Humidity ( %RH )"() -> (w2137:dbl)
                    "Humidity ( %RH )" <- w2137
                    "Humidity ( %RH )" <- w2137
                    n775 = local read "TEMP"() -> (w2138:dbl)
                    "Temp" <- w2138
                    "Temperature ( Deg C )" <- w2138
                    n776 = local write "FF 3"(w2139) -> ()
                    n777 = local read "ecr"() -> (w2135:dbl)
                    "ecr 2" <- w2135
                    "Electrical Contact Resistance ( % )" <- w2135
                    "ecr 4" <- w2135
                    n778 = Multiply(x=w2150, y=0.05) -> (x*y=w2152:dbl)
                    n779 = local read "COF 2"() -> (w2140:dbl)
                    "cof" <- w2140
                    "Coefficient of Friction" <- w2140
                    "COF 4" <- w2140
                    "Coefficient of Friction" <- w2140
                    n780 = local read "Frequency ( Hz )"() -> (w2146:dbl)
                    n781 = local write "ecr 3"(w2135) -> ()
                    n782 = Add(x=w2152, y=w2153) -> (x+y=w2134:dbl)
                    "Stroke Ln" <- w2134
                    "Stroke 2" <- w2134
                    "Disp" <- w2134
                    "Stroke 3" <- w2134
                    "Stroke 4" <- w2134
                    n783 = Bundle("y"=1.02, w2134, "y"=0.08) -> (→"Stroke ( mm )" →"Stroke ( mm )":cluster{"y":dbl, dbl, "y":dbl})  [unwired: 1 in]
                    n784 = local write "Temperature ( Deg C )"(w2138) -> ()
                    n785 = local read "Elapsed time"() -> (w2178:dbl)
                    n786 = local read "AIR TEMP"() -> (w2143:dbl)
                    n787 = local write "Electrical Contact Resistance ( % )"(w2135) -> ()
                    n788 = local write "COF 3"(w2140) -> ()
                    n789 = local read "PID-out"() -> (w2149:dbl)
                    n790 = Number To Fractional String(number=w2140, width (-)=i16 9 ("precision (6)"), precision (6)=i16 6) -> (F-format string=w2179:string)  [unwired: 1 in]
                    n791 = Number To Fractional String(number=w2134, width (-)=i16 9 ("precision (6)"), precision (6)=i16 6) -> (F-format string=w2171:string)  [unwired: 1 in]
                    n792 = Number To Fractional String(number=w2143, width (-)=i16 9 ("precision (6)"), precision (6)=i16 3) -> (F-format string=w2170:string)  [unwired: 1 in]
                    n793 = Number To Fractional String(number=w2138, width (-)=i16 9 ("precision (6)"), precision (6)=i16 3) -> (F-format string=w2167:string)  [unwired: 1 in]
                    n794 = Number To Fractional String(number=w2137, width (-)=i16 9 ("precision (6)"), precision (6)=i16 3) -> (F-format string=w2164:string)  [unwired: 1 in]
                    n795 = Number To Fractional String(number=w2135, width (-)=i16 9 ("precision (6)"), precision (6)=i16 3) -> (F-format string=w2160:string)  [unwired: 1 in]
                    n796 = Number To Fractional String(number=w2149, width (-)=i16 9 ("precision (6)"), precision (6)=i16 3) -> (F-format string=w2155:string)  [unwired: 1 in]
                    n797 = Number To Fractional String(number=w2146, width (-)=i16 9 ("precision (6)"), precision (6)=i16 3) -> (F-format string=w2145:string)  [unwired: 1 in]
                    n798 = Number To Fractional String(number=w2178, width (-)=i16 14 ("precision (6)"), precision (6)=i16 3) -> (F-format string=w2180:string)  [unwired: 1 in]
                    n799 = local read "FILE"() -> (w2186:string)
                    n800 = Concatenate Strings("C:\\LAB-IQ-NXT\\Data\\" ("string"), w2186, ".dgf" ("Substring")) -> (w2188:string)
                    n801 = String To Path(string=w2188) -> (path=w2187:path)
                    n802 = Concatenate Strings(w2180, w2154, w2179, w2154, w2171, w2154, w2170, w2154, w2167, w2154, w2164, w2154, w2160, w2154, w2155, w2154, w2145, "\r") -> (w2177:string)
                    n803 = call <vilib>:"Write Characters To File.vi"("append to file? (new file:F)"=TRUE, "character string"=w2177, "file path (dialog if empty)"=w2187) -> ()  [unwired: 2 in, 1 out]
                    "refresh flag" <- TRUE ("refresh flag")
                  }
                }
                n804 = local read "COUNT"() -> (w2092:i32)
                n805 = Multiply(x=w2106, y=w2092) -> (x*y=w2098:dbl)
                n806 = Add(x=w2101, y=w2098) -> (x+y=w2085:dbl)
                "Elapsed time 3" <- w2085
                n807 = local read "Test \nStatus"() -> (w2086:bool)
                n808 = local read "clk"() -> (w2093:dbl)
                n809 = Equal?(x=w2093, y=10.0) -> (x = y?=w2095:bool)
                n810 = Divide(x=w2085, y=60.0) -> (x/y=w2096:dbl)
                n811 = case shown="True" w2086 {
                  tunnel: w2096 -> [_ w2118]
                  tunnel: w2101 -> [_ w2126]
                  tunnel: [0.0 w2122] -> _
                  tunnel: w2095 -> [_ w2121]
                  tunnel: [0.0 w2120] -> _
                  tunnel: w2085 -> [_ w2120]
                  tunnel: w2099 -> [w2114 _]
                  frame False {
                    n812 = local write "acq timer"(w2114) -> ()
                  }
                  frame True {
                    n813 = local read "Set Hz"() -> (w2123:dbl)
                    n814 = local write "Elapsed time"(w2118) -> ()
                    n815 = local read "test time"() -> (w2119:dbl)
                    n816 = Multiply(x=w2126, y=w2123) -> (x*y=w2125:dbl)
                    n817 = case shown="False" w2121 {
                      tunnel: w2125 -> [w2127 _]
                      tunnel: [w2127 1.0] -> w2122
                      frame False {
                        n818 = local write "Cycles elapsed"(w2127) -> ()
                      }
                      frame True {
                      }
                    }
                    n819 = Subtract(x=w2119, y=w2118) -> (x-y=w2117:dbl)
                    "time" <- w2117
                    n820 = Greater?(x=w2118, y=w2119) -> (0:w2124:bool)
                    n821 = case shown="True" w2124 {
                      frame False {
                      }
                      frame True {
                        n822 = local read "Humidity ( %RH )"() -> (→"Rh After":dbl)
                        n823 = property on="STOP 2" class="Bool (strict)"("Disabled"=u8 0) -> ()  [unwired: 2 in, 2 out]
                        n824 = local write "RUN"(FALSE ("OK Button 2")) -> ()
                        n825 = local write "STOP 3"(TRUE ("STOP")) -> ()
                      }
                    }
                    n826 = local write "Time Remaining"(w2117) -> ()
                  }
                }
              }
              frame #2 {
                n827 = case shown="True" "Heater Button" {
                  tunnel: [0.0 ("output") w2212] -> w2191
                  frame False {
                    w2193 = TRUE ("tmpchk")
                    n828 = local write "tmpchk"(w2193) -> ()
                    n829 = local write "Reset 4"(w2193) -> ()
                    n830 = local read "TEMP"() -> (w2194:dbl)
                    n831 = local write "Temp ini"(w2194) -> ()
                    n832 = local write "reinit"(TRUE ("reinit")) -> ()
                  }
                  frame True {
                    # "Logic to turn off\nthe heater when \ntemp is not rising.\nTime - 60 sec\nDelta t- 5°c"
                    n833 = local read "Set Temp"() -> (w2209:dbl)
                    n834 = local read "Temp ini"() -> (w2200:dbl)
                    n835 = local read "TEMP"() -> (w2203:dbl)
                    n836 = Add(x=w2209, y=0.5) -> (x+y=w2207:dbl)
                    n837 = Less?(x=w2200, y=53.0) -> (x < y?=w2198:bool)
                    n838 = Greater Or Equal?(x=w2203, y=w2207) -> ()  [unwired: 1 out]
                    n839 = And(x="tmpchk", y=w2198) -> (x .and. y?=w2201:bool)
                    n840 = case shown="True" w2201 {
                      frame False {
                      }
                      frame True {
                        n841 = call "Elapsed Time8"("Time Target (s)"=300.0, "Reset"="Reset 4") -> ("Time has Elapsed"=w2217:bool)  [unwired: 10 in, 7 out]
                        n842 = flat-sequence {
                          tunnel: w2217 -> [_]
                          frame #0 {
                            n843 = local write "Reset 4"(FALSE ("Reset 4")) -> ()
                          }
                        }
                        n844 = case shown="True" w2217 {
                          frame False {
                          }
                          frame True {
                            n845 = local read "Temp ini"() -> (w2224:dbl)
                            n846 = local read "TEMP"() -> (w2225:dbl)
                            n847 = Add(x=w2224, y=5.0) -> (x+y=w2222:dbl)
                            n848 = Greater?(x=w2225, y=w2222) -> (0:w2223:bool)
                            n849 = case shown="False" w2223 {
                              frame False {
                                n850 = local write "Heater Button"(FALSE ("Heater Button")) -> ()
                              }
                              frame True {
                                n851 = local write "tmpchk"(FALSE ("tmpchk")) -> ()
                              }
                            }
                          }
                        }
                      }
                    }
                    n852 = call-poly <vilib>:"PID.vi"("reinitialize? (F)"="reinit", "output range"="output range", "dt (s)"=-1.0, "PID gains"="Temp PID gains", "process variable"=w2203, "setpoint"=w2209) -> ("output"=w2206:dbl)  [unwired: 4 in, 1 out]
                    n853 = Select(t=0.0, s=FALSE, f=w2206) -> (s? t:f=w2205:dbl)
                    "PID output" <- w2205
                    n854 = Subtract(x=w2209, y=w2203) -> (x-y=w2211:dbl)
                    n855 = flat-sequence {
                      tunnel: w2205 -> [w2228]
                      tunnel: [w2228] -> w2212
                      frame #0 {
                        n856 = local write "reinit"(FALSE ("reinit")) -> ()
                      }
                    }
                    n857 = Bundle(w2211, "output"=w2205, "TEMP"=w2203) -> (→"gTEMP 3":cluster{dbl, "output":dbl, "TEMP":dbl})  [unwired: 1 in]
                  }
                }
                "PID-out" <- w2191
              }
              frame #3 {
                n858 = local read "TEMP"() -> (w2230:dbl)
                n859 = Greater Or Equal?(x=w2230, y="Set Temp 2") -> (x >= y?=w2235:bool)
                n860 = case shown="True" w2235 {
                  tunnel: [FALSE TRUE] -> w2233
                  frame False {
                  }
                  frame True {
                  }
                }
                "Status 13" <- w2233
                n861 = And(x=w2233, y="trip1 8") -> (x .and. y?=w2232:bool)
                n862 = case shown="True" w2232 {
                  frame False {
                  }
                  frame True {
                    w2236 = FALSE ("OK Button 2")
                    n863 = local write "Heater Button"(w2236) -> ()
                    n864 = local write "RUN"(w2236) -> ()
                  }
                }
              }
            }
          }
        }
        n865 = stacked-sequence {
          frame #0 {
            n866 = case shown="True" "RST FF" {
              frame False {
              }
              frame True {
                w1974 = 0.0 ("X Scale.Range:Maximum")
                n867 = property on="Frictional Force ( N )" class="WFChart (strict)"("XScale.Maximum"=600.0 ("X Scale.Range:Maximum"), "XScale.Minimum"=w1974, "YScale.Maximum"=10.0 ("Y Scale.Range:Maximum"), "YScale.Minimum"=w1974) -> ()  [unwired: 2 in, 2 out]
              }
            }
          }
          frame #1 {
            n868 = case shown="True" "RST TEMP" {
              frame False {
              }
              frame True {
                n869 = property on="Temperature ( Deg C )" class="WFChart (strict)"("XScale.Minimum"=0.0 ("X Scale.Range:Minimum"), "XScale.Maximum"=600.0 ("X Scale.Range:Maximum"), "YScale.Minimum"=0.0 ("Y Scale.Range:Minimum"), "YScale.Maximum"=100.0 ("Y Scale.Range:Maximum")) -> ()  [unwired: 2 in, 2 out]
              }
            }
          }
          frame #2 {
            n870 = case shown="True" "RSTCOF" {
              frame False {
              }
              frame True {
                n871 = property on="Coefficient of Friction" class="WFChart (strict)"("XScale.Minimum"=0.0 ("X Scale.Range:Minimum"), "XScale.Maximum"=600.0 ("X Scale.Range:Maximum"), "YScale.Maximum"=1.0 ("X Scale.Range:Minimum"), "YScale.Minimum"=0.0 ("X Scale.Range:Minimum")) -> ()  [unwired: 2 in, 2 out]
              }
            }
          }
          frame #3 {
            n872 = case shown="True" "RSTCOF 2" {
              frame False {
              }
              frame True {
                (unwired) 100.0 ("Y Scale.Range:Maximum")
                (unwired) 0.0 ("Y Scale.Range:Minimum")
                (unwired) 600.0 ("X Scale.Range:Maximum")
                (unwired) 0.0 ("X Scale.Range:Minimum")
              }
            }
          }
          frame #4 {
            n873 = case shown="True" "RSTCOF 3" {
              frame False {
              }
              frame True {
                n874 = property on="Electrical Contact Resistance ( % )" class="WFChart (strict)"("XScale.Minimum"=0.0 ("X Scale.Range:Minimum"), "XScale.Maximum"=600.0 ("X Scale.Range:Maximum"), "YScale.Minimum"=0.0 ("Y Scale.Range:Minimum"), "YScale.Maximum"=100.0 ("Y Scale.Range:Maximum")) -> ()  [unwired: 2 in, 2 out]
              }
            }
          }
        }
        n875 = disable-structure shown="Disabled" {
          frame Disabled {
            n876 = case shown="True" {
              selector: _ -> [_ _]
              frame False {
              }
              frame True {
                w1907 = TRUE ("Heater")
                n877 = local write "Humidity"(w1907) -> ()
                n878 = local write "Heater Button"(w1907) -> ()
                n879 = local read "TEST STANDARD"() -> (w1910:T3)
                n880 = local read "TEST STANDARD"() -> (w1905:T3)
                n881 = Equal?(x=w1910, y=enum16{"ASTM D6079", "ISO 12156", "Custom"}."ISO 12156" ("Test Standard")) -> (x = y?=w1908:bool)
                n882 = Equal?(x=w1905, y=enum16{"ASTM D6079", "ISO 12156", "Custom"}."ASTM D6079" ("Test Standard")) -> (x = y?=w1904:bool)
                n883 = case shown="True" w1908 {
                  frame False {
                  }
                  frame True {
                    n884 = local write "airtempflg"(FALSE ("airtempflg")) -> ()
                    n885 = local write "Heater"(TRUE ("Heater")) -> ()
                  }
                }
                n886 = case shown="True" w1904 {
                  frame False {
                  }
                  frame True {
                    n887 = local write "airtempflg"(TRUE ("airtempflg")) -> ()
                    n888 = local write "Heater"(FALSE ("Heater")) -> ()
                  }
                }
              }
            }
          }
          frame Enabled {
          }
        }
        n889 = local read "RUN"() -> (w1862:bool)
        n890 = case shown="True" w1862 {
          tunnel: [FALSE ("TEST RUNNING") TRUE ("TEST RUNNING")] -> w1853
          frame False {
            w1995 = 0.0 ("Flag")
            n891 = local write "Flag"(w1995) -> ()
            n892 = local write "Time Remaining"(w1995) -> ()
            n893 = local write "Elapsed time"(0.0 ("elapsedtime")) -> ()
          }
          frame True {
            n894 = local write "Flag"(10.0 ("Flag")) -> ()
          }
        }
        n895 = local read "Flag"() -> (w1859:dbl)
        n896 = local read "RUN"() -> (w1856:bool)
        n897 = Equal?(x=w1859, y=10.0) -> (x = y?=w1857:bool)
        n898 = Not(x=w1856) -> (.not. x?=w1855:bool)
        n899 = And(x=w1857, y=w1855) -> (x .and. y?=w1854:bool)
        n900 = case shown="True" w1854 {
          frame False {
          }
          frame True {
            w1972 = FALSE ("Heater Button")
            n901 = local write "Heater Button"(w1972) -> ()
            n902 = local write "Humidity"(w1972) -> ()
          }
        }
        n903 = local write "Save"(w1853) -> ()
        n904 = local write "Test \nStatus"(w1853) -> ()
        n905 = local write "st enable"(w1853) -> ()
        n906 = local write "PWR"(w1853) -> ()
        n907 = local read "Set Temp"() -> (w1815:dbl)
        n908 = local read "SetTemp"() -> (w1817:dbl)
        n909 = local read "Set Rh"() -> (w1816:dbl)
        n910 = local read "Amb temp"() -> (w1814:dbl)
        n911 = local read "Humidity ( %RH )"() -> (w1813:dbl)
        n912 = local read "TEMP"() -> (w1812:dbl)
        n913 = Add(x=w1817, y=w1842) -> (x+y=w1843:dbl)
        n914 = Subtract(x=w1817, y=w1842) -> (x-y=w1844:dbl)
        n915 = Add(x=w1816, y=w1841) -> (x+y=w1840:dbl)
        n916 = Subtract(x=w1816, y=w1841) -> (x-y=w1839:dbl)
        n917 = Add(x=w1815, y=w1836) -> (x+y=w1837:dbl)
        n918 = Subtract(x=w1815, y=w1836) -> (x-y=w1838:dbl)
        n919 = In Range and Coerce(upper limit=w1843, x=w1814, lower limit=w1844) -> (In Range?=w1833:bool)  [unwired: 1 out]
        n920 = In Range and Coerce(upper limit=w1840, x=w1813, lower limit=w1839) -> (In Range?=w1831:bool)  [unwired: 1 out]
        n921 = In Range and Coerce(upper limit=w1837, x=w1812, lower limit=w1838) -> (In Range?=w1829:bool)  [unwired: 1 out]
        n922 = case shown="True" w1833 {
          tunnel: [FALSE ("RUN") TRUE ("RUN")] -> w1832
          tunnel: [_ 1] -> w1825
          frame False {
          }
          frame True {
          }
        }
        n923 = case shown="True" w1831 {
          tunnel: [FALSE ("RUN") TRUE ("RUN")] -> w1830
          tunnel: [_ 2] -> w1824
          frame False {
          }
          frame True {
          }
        }
        n924 = case shown="True" w1829 {
          tunnel: [FALSE ("RUN") TRUE ("RUN")] -> w1828
          tunnel: [_ 3] -> w1823
          frame False {
          }
          frame True {
          }
        }
        n925 = local read "airtempflg"() -> (w1834:bool)
        n926 = Or(x=w1834, y=w1832) -> (x .or. y?=w1835:bool)
        n927 = Build Array(w1825, w1824, w1823) -> (w1821:i32[])
        n928 = disable-structure shown="Disabled" {
          disable-tunnel: w1835 -> [w1868 _]
          disable-tunnel: w1830 -> [w1867 _]
          disable-tunnel: w1828 -> [w1866 _]
          frame Disabled {
            n929 = Compound Arithmetic op=AND(w1868, w1867, w1866) -> ()  [unwired: 1 out]
            n930 = case shown="True" {
              selector: _ -> [_ _]
              frame False {
              }
              frame True {
